vi "Get JSON Data.vi"(7 "Panel Origin":T1, 8 "error in (no error)":errorcluster, 9 "Force Get All Data":bool, 10 "VI Reference":refnum<vi>, 11 "Progress In":refnum<class "Progressbar.lvclass">) -> (0 "error out":errorcluster, 2 "JSON string":string, 3 "Progress Out":refnum<class "Progressbar.lvclass">)   [LabVIEW 2015, in "Front Panel Publisher.lvlib" / "Progressbar.lvclass"]
uses:
  Progressbar.lvclass
  <vilib>/Utility/miscctls.llb/LVPointTypeDef.ctl
  Text_class/Text.lvclass
  Control_class/Control.lvclass
  Object_class/Object.lvclass
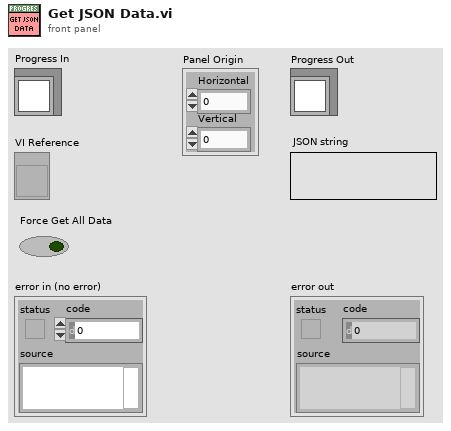
[diagram p1: front panel]
types:
  T1 = typedef "LVPointTypeDef.ctl" = cluster{"Horizontal":i16, "Vertical":i16}
  T2 = typedef "Front Panel Publisher.lvlib/Progressbar.lvclass/Attributes.ctl" = cluster{"Maximum":dbl, "Minimum":dbl}
  T3 = typedef "Front Panel Publisher.lvlib/Object.lvclass/Attributes.ctl" = cluster{"UID":i32, "Type":string, "Coordinates":T4, "Reference":refnum<vi>}
  T4 = typedef "Front Panel Publisher.lvlib/Object.lvclass/Coordinates.ctl" = cluster{"Left":i32, "Top":i32, "Height":u32, "Width":u32}
  T5 = typedef "Front Panel Publisher.lvlib/Control.lvclass/Attributes.ctl" = cluster{"Description":string, "Indicator":bool, "Default Value":variant, "Control Index":i32, "Label":refnum<class "Text.lvclass">, "Caption":refnum<class "Text.lvclass">, "Image b64":string, "Use Picture":bool, "Value Only":bool}
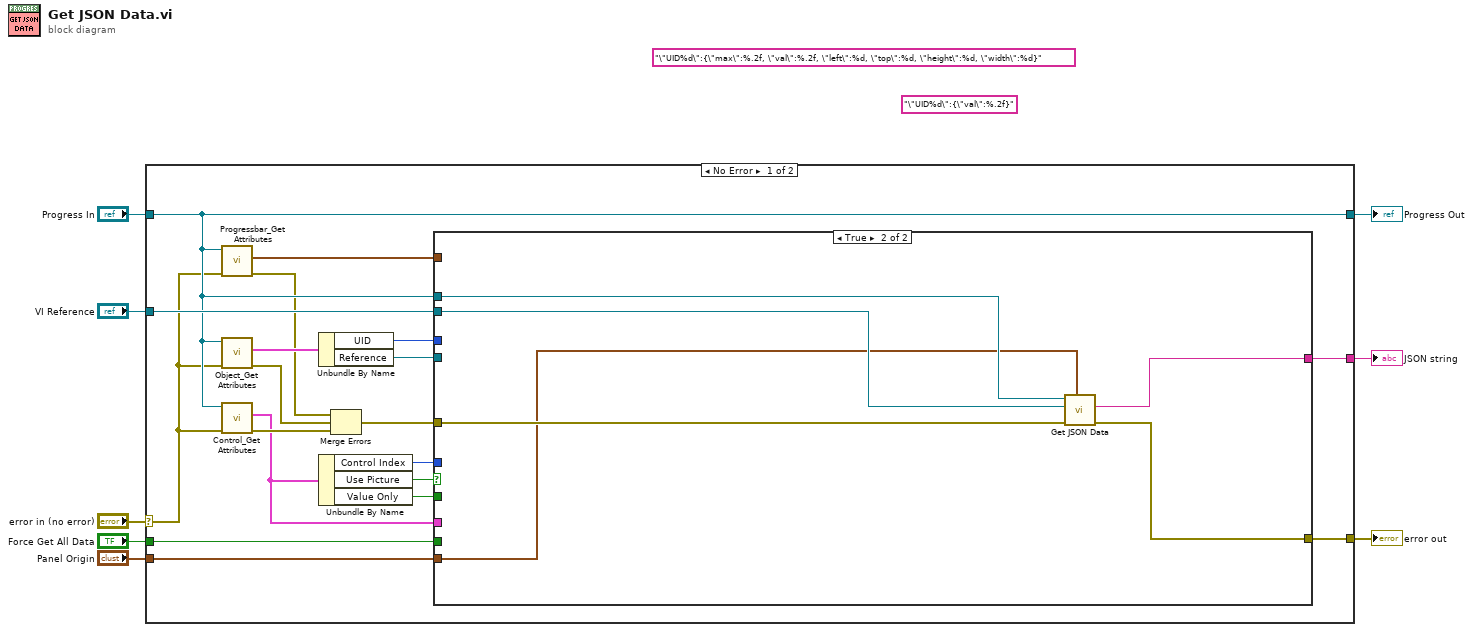
[diagram p0: block diagram]
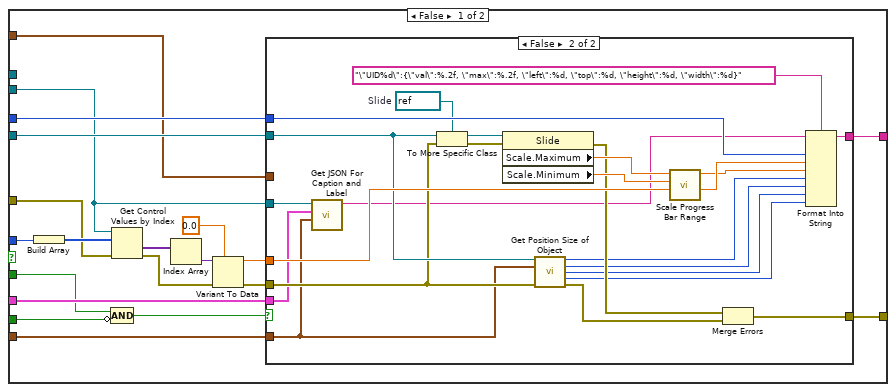
[diagram p2: hidden frame]
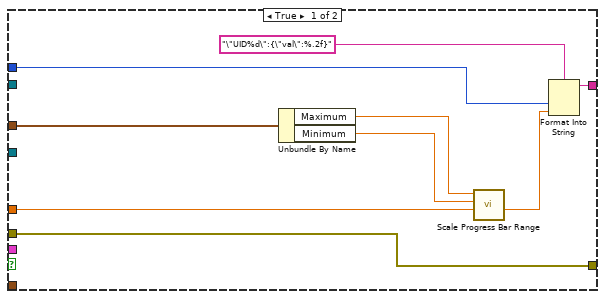
[diagram p3: hidden frame]
diagram:
  (unwired) "\"UID%d\":{\"val\":%.2f}"
  (unwired) "\"UID%d\":{\"max\":%.2f, \"val\":%.2f, \"left\":%d, \"top\":%d, \"height\":%d, \"width\":%d}"
  n1 = case shown="No Error" "error in (no error)" {
    selector: "error in (no error)" -> [w14 w88]
    tunnel: [w22 w88] -> w7
    tunnel: [w15 w87] -> w5
    tunnel: "Progress In" -> [w15 w87]
    tunnel: "VI Reference" -> [w18 _]
    tunnel: [w26 _] -> w3
    tunnel: "Force Get All Data" -> [w10 _]
    tunnel: "Panel Origin" -> [w9 _]
    frame No Error {
      n2 = call "Progressbar_Get Attributes.vi"("error in (no error)"=w14, "Progress In"=w15) -> ("error out"=w13:errorcluster, "Data"=w12:T2)  [unwired: 6 in, 2 out]
      n3 = call "Object_Get Attributes.vi"("error in (no error)"=w14, "Object In"=w15) -> ("error out"=w27:errorcluster, "Data"=w25:T3)  [unwired: 6 in, 2 out]
      n4 = call "Control_Get Attributes.vi"("error in (no error)"=w14, "Control In"=w15) -> ("error out"=w20:errorcluster, "Data"=w11:T5)  [unwired: 6 in, 2 out]
      n5 = Unbundle By Name(w25) -> ("UID"=w24:i32, "Reference"=w23:refnum<vi>)
      n6 = Unbundle By Name(w11) -> ("Control Index"=w17:i32, "Use Picture"=w19:bool, "Value Only"=w16:bool)
      n7 = Merge Errors(w13, w27, w20) -> (w21:errorcluster)
      n8 = case shown="True" w19 {
        tunnel: [w47 w82] -> w26
        tunnel: w24 -> [w46 _]
        tunnel: w23 -> [w45 _]
        tunnel: [w37 w83] -> w22
        tunnel: w21 -> [w36 w84]
        tunnel: w18 -> [w33 w85]
        tunnel: w15 -> [_ w86]
        tunnel: w17 -> [w39 _]
        tunnel: w16 -> [w30 _]
        tunnel: w12 -> [w34 _]
        tunnel: w11 -> [w32 _]
        tunnel: w10 -> [w31 _]
        tunnel: w9 -> [w28 w81]
        frame False {
          n9 = Build Array(w39) -> (w43:i32[])
          n10 = Compound Arithmetic op=AND(w30, invert w31) -> (w29:bool)
          n11 = Get Control Values by Index(0:w33, 1:w43, 3:w36) -> (10:w42:variant[], 11:w44:errorcluster)
          n12 = Index Array(array=w42) -> (element=w41:variant)  [unwired: 1 in]
          n13 = Variant To Data(error in=w44, type=0.0, Variant=w41) -> (data=w38:dbl, error out=w35:errorcluster)
          n14 = case shown="False" w29 {
            tunnel: [w55 w79] -> w47
            tunnel: w46 -> [w54 w78]
            tunnel: w45 -> [_ w71]
            tunnel: w38 -> [w52 w73]
            tunnel: [w51 w68] -> w37
            tunnel: w35 -> [w51 w70]
            tunnel: w34 -> [w50 _]
            tunnel: w33 -> [_ w62]
            tunnel: w32 -> [_ w61]
            tunnel: w28 -> [_ w57]
            frame True {
              n15 = Unbundle By Name(w50) -> ("Maximum"=w49:dbl, "Minimum"=w48:dbl)
              n16 = call "Scale Progress Bar Range.vi"("Value"=w52, "Minimum"=w48, "Maximum"=w49) -> ("Value Out"=w53:dbl)  [unwired: 7 in, 1 out]
              n17 = Format Into String(format string="\"UID%d\":{\"val\":%.2f}", w54, w53) -> (resulting string=w55:string)  [unwired: 2 in, 1 out]
            }
            frame False {
              w76 = refnum<vi> refnum  # Slide
              n18 = call "Get JSON For Caption and Label.vi"("Panel Origin"=w57, "Data"=w61, "VI in"=w62) -> ("JSON"=w60:string)  [unwired: 7 in, 1 out]
              n19 = To More Specific Class(target class=w76, reference=w71, error in=w70) -> (specific class reference=w77:refnum<vi>, error out=w80:errorcluster)
              n20 = property class="Slide"(reference=w77, error in=w80) -> (error out=w72:errorcluster, "Scale.Maximum"=w74:dbl, "Scale.Minimum"=w75:dbl)  [unwired: 1 out]
              n21 = call "Get Position Size of Object.vi"("GObject in"=w71, "Panel Origin"=w57, "error in (no error)"=w70) -> ("Left"=w66:i32, "Top"=w65:i32, "Height"=w64:u32, "Width"=w63:u32, "error out"=w67:errorcluster)  [unwired: 8 in]
              n22 = call "Scale Progress Bar Range.vi"("Value"=w73, "Minimum"=w75, "Maximum"=w74) -> ("Value Out"=w59:dbl, "Maximum Out"=w58:dbl)  [unwired: 7 in]
              n23 = Merge Errors(w72, w67) -> (w68:errorcluster)
              n24 = Format Into String(format string="\"UID%d\":{\"val\":%.2f, \"max\":%.2f, \"left\":%d, \"top\":%d, \"height\":%d, \"width\":%d}", initial string=w60, w78, w59, w58, w66, w65, w64, w63) -> (resulting string=w79:string)  [unwired: 1 in, 1 out]
            }
          }
        }
        frame True {
          n25 = call-parent "Get JSON Data.vi"("Panel Origin"=w81, "error in (no error)"=w84, "VI Reference"=w85, "Control In"=w86) -> ("error out"=w83:errorcluster, "JSON string"=w82:string)  [unwired: 5 in, 1 out]
        }
      }
    }
    frame Error {
    }
  }
  "error out" <- w7
  "Progress Out" <- w5
  "JSON string" <- w3
